vi "CAN 6 SPARK MAX Motor Get Encoder.vi"(7 "Distance per tick":dbl=0.012118448224296566 format="%#_13g", 11 "Drivetrain":T2) -> (3 "Position":cluster{dbl, dbl})   [LabVIEW 2018]
uses:
  <vilib>/Rock Robotics/SystemInterfaces/DIO/FPGA_DIOPWMChannel.ctl
  <vilib>/Rock Robotics/WPI/PWM/WPI_PWMDeadband.ctl
  <vilib>/Rock Robotics/WPI/MotorControl/WPI_MotorControlType.ctl
  <vilib>/Rock Robotics/SystemInterfaces/DIO/FPGA_DIOChannel.ctl
  <vilib>/Rock Robotics/WPI/MotorControl/WPI_MotorControlDeviceRef.ctl
  SPARKMAX6Motor.ctl
panel:
  out "Velocity (RPM)":T1
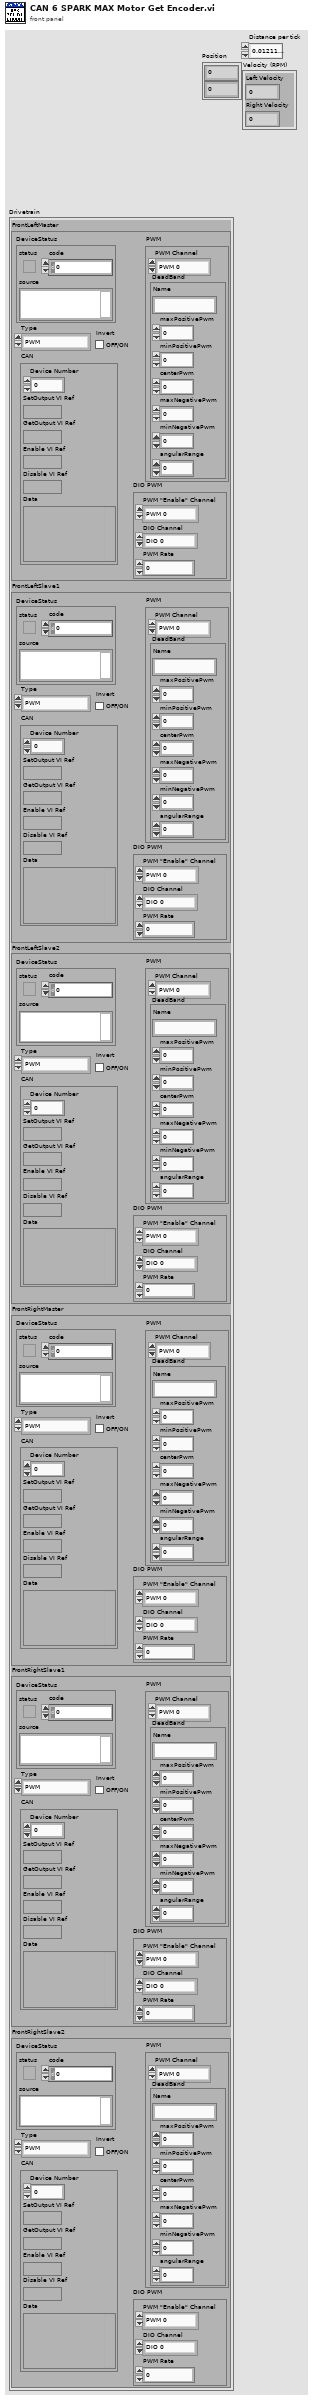
[diagram p1: front panel]
types:
  T1 = cluster{"Left Velocity":dbl, "Right Velocity":dbl}
  T2 = typedef "SPARKMAX6Motor.ctl" = cluster{"FrontLeftMaster":T3, "FrontLeftSlave1":T3, "FrontLeftSlave2":T3, "FrontRightMaster":T3, "FrontRightSlave1":T3, "FrontRightSlave2":T3}
  T3 = typedef "WPI_MotorControlDeviceRef.ctl" = cluster{"DeviceStatus":errorcluster, "Type":T4, "PWM":cluster{"PWM Channel":T5, "DeadBand":T6}, "CAN":cluster{"Device Number":u8, "SetOutput VI Ref":variant, "GetOutput VI Ref":variant, "Enable VI Ref":variant, "Disable VI Ref":variant, "Data":variant}, "Invert":bool, "DIO PWM":cluster{"PWM \"Enable\" Channel":T5, "DIOChannel":T7, "PWM Rate":dbl}}
  T4 = typedef "WPI_MotorControlType.ctl" = enum16{"PWM", "CAN", "DIO PWM"}
  T5 = typedef "FPGA_DIOPWMChannel.ctl" = enum8{"PWM 0", "PWM 1", "PWM 2", "PWM 3", "PWM 4", "PWM 5", "PWM 6", "PWM 7", "PWM 8", "PWM 9", "PWM MXP 0", "PWM MXP 1", "PWM MXP 2", "PWM MXP 3", "PWM MXP 4", "PWM MXP 5", "PWM MXP 6", "PWM MXP 7", "PWM MXP 8", "PWM MXP 9", "Invalid"}
  T6 = typedef "WPI_PWMDeadband.ctl" = cluster{"Name":string, "maxPositivePwm":i32, "minPositivePwm":i32, "centerPwm":i32, "maxNegativePwm":i32, "minNegativePwm":i32, "angularRange":u16}
  T7 = typedef "FPGA_DIOChannel.ctl" = enum8{"DIO 0", "DIO 1", "DIO 2", "DIO 3", "DIO 4", "DIO 5", "DIO 6", "DIO 7", "DIO 8", "DIO 9", "DIO MXP 0", "DIO MXP 1", "DIO MXP 2", "DIO MXP 3", "DIO MXP 4", "DIO MXP 5", "DIO MXP 6", "DIO MXP 7", "DIO MXP 8", "DIO MXP 9", "DIO MXP 10", "DIO MXP 11", "DIO MXP 12", "DIO MXP 13", "DIO MXP 14", "DIO MXP 15", "SPI Port CS1", "SPI Port CS2", "SPI Port CS3", "SPI Port MISO", "SPI Port MOSI", "Invalid"}
  T8 = cluster{"Sensor Velocity":dbl, "Sensor Velocity":dbl}
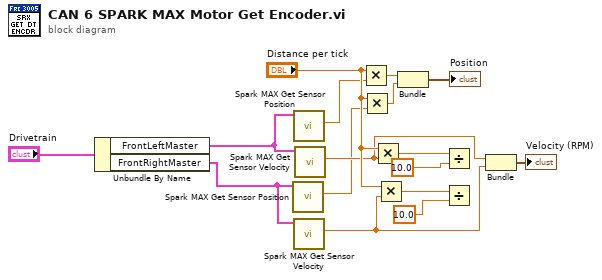
[diagram p0: block diagram]
diagram:
  n1 = Unbundle By Name("Drivetrain") -> ("FrontLeftMaster"=w5:T3, "FrontRightMaster"=w2:T3)
  n2 = call <vilib>:"Spark MAX Get Sensor Position.vi"("MotorControlDevRef in"=w2) -> ("Sensor Position"=w4:dbl)  [unwired: 7 in, 3 out]
  n3 = call <vilib>:"Spark MAX Get Sensor Position.vi"("MotorControlDevRef in"=w5) -> ("Sensor Position"=w7:dbl)  [unwired: 7 in, 3 out]
  n4 = call <vilib>:"Spark MAX Get Sensor Velocity.vi"("MotorControlDevRef in"=w2) -> ("Sensor Velocity"=w3:dbl)  [unwired: 7 in, 3 out]
  n5 = call <vilib>:"Spark MAX Get Sensor Velocity.vi"("MotorControlDevRef in"=w5) -> ("Sensor Velocity"=w6:dbl)  [unwired: 7 in, 3 out]
  n6 = Multiply(x="Distance per tick", y=w7) -> (x*y=w16:dbl)
  n7 = Multiply(x="Distance per tick", y=w4) -> (x*y=w14:dbl)
  n8 = Multiply(x="Distance per tick", y=w6) -> (x*y=w12:dbl)
  n9 = Multiply(x="Distance per tick", y=w3) -> (x*y=w10:dbl)
  n10 = Bundle(w16, w14) -> (→"Position":cluster{dbl, dbl})  [unwired: 1 in]
  n11 = Divide(x=w12, y=10.0) -> ()  [unwired: 1 out]
  n12 = Divide(x=w10, y=10.0) -> ()  [unwired: 1 out]
  n13 = Bundle("Sensor Velocity"=w6, "Sensor Velocity"=w3) -> (→"Velocity (RPM)":T8)  [unwired: 1 in]
